vi "Message Window Dialog Box.vi"(4 "parent window name (\"\")":string, 5 "sound? (F)":bool, 6 "modality (0)":i32(ring) items=["Application", "System", "Task"], 7 "icon (0:None)":i32(ring), 8 "buttons (0:OK)":i32(ring), 9 "message (\"\")":string, 10 "window title (\"\")":string) -> (3 "button pressed":i32(ring) items=["OK", "CANCEL", "ABORT", "RETRY", "IGNORE", "YES", "NO"])   [LabVIEW 2011]
doc: "This VI calls the Windows functions MessageBox and MessageBeep to display a message dialog box and, optionally, play a sound effect. These functions are in the Windows DLL called USER.EXE, which is located in the windows\\system directory. If your computer is not equipped with a sound driver, a short \"beep\" will be played through the PC's speaker.\n\nVarious combinations of dialog boxes are possible. The buttons input selects which buttons are displayed in the dialog box, the icon input determines the icon, if any, and the modality box determines whether the dialog box is system, application, or task modal.\n\nThe following dialog box button schemes are available through the \"buttons\" input:\n0: OK\n1: OK / Cancel\n2: Abort / Retry / Ignore\n3: Yes / No / Cancel\n4: Yes / No\n5: Retry / Cancel\n\nThe following icons are available through the \"icon\" input:\n0: None\n1: STOP icon\n2: Question icon\n3: Exclamation icon\n4: Information icon\n\nThe following three modalities are available:\n0: Application\n1: System\n2: Task\n\nIf sounds are enabled, the icon option determines the sound effect played, as defined in the Sounds section of Windows' Control Panel.\n\nThe DLL functions called are:\n\nint MessageBox ( hWndParent, lpText, lpCaption, wType )\nvoid MessageBeep ( wType )\n\nFunction definitions are from:\nMicrosoft Windows Programmer's Reference\nCopyright 1990 Microsoft Corporation."
uses:
  user32.dll
panel:
  in  "buttons":i32[](array[numeric])=[0, 1, 2, 3, 4, 5, 16, 32, 48, 64] format="%.0x"
  in  "icons":i32[](array[numeric])=[0, 16, 32, 48, 64, 5, 16, 32, 48, 64] format="%.0x"
  in  "modal constants":i32[](array[numeric])=[0, 4096, 8192] format="%.0x"
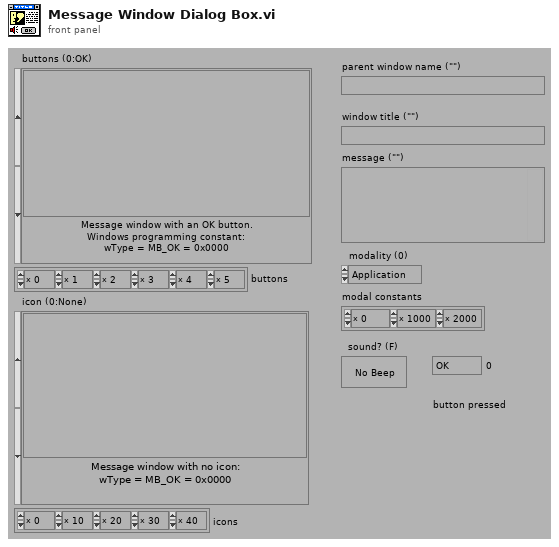
[diagram p1: front panel]
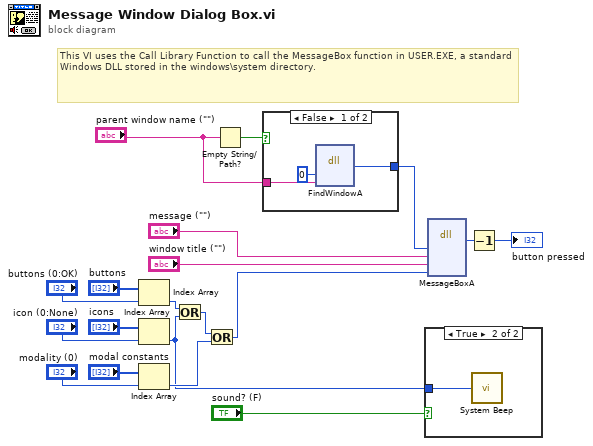
[diagram p0: block diagram]
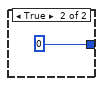
[diagram p2: hidden frame]
diagram:
  # "This VI uses the Call Library Function to call the MessageBox function in USER.EXE, a standard Windows DLL stored in the windows\\system directory."
  n1 = Index Array(array="buttons", index="buttons (0:OK)") -> (element=w7:i32)
  n2 = Index Array(array="icons", index="icon (0:None)") -> (element=w4:i32)
  n3 = Index Array(array="modal constants", index="modality (0)") -> (element=w6:i32)
  n4 = Or(x=w7, y=w4) -> (x .or. y?=w5:i32)
  n5 = Or(x=w5, y=w6) -> (x .or. y?=w11:i32)
  n6 = Empty String/Path?(string/path="parent window name (\"\")") -> (empty?=w2:bool)
  n7 = case shown="False" w2 {
    tunnel: [w21 u32 0] -> w3
    tunnel: "parent window name (\"\")" -> [w20 _]
    frame False {
      n8 = dll-call lib="User32.dll" fn="FindWindowA" label="FindWindow"("lpszClassName"=0, "lpszWindowName"=w20) -> ("hWnd"=w21:u32)  [unwired: 5 in, 2 out]
    }
    frame True {
    }
  }
  n9 = case shown="True" "sound? (F)" {
    tunnel: w4 -> [_ w24]
    frame False {
      # "Do not play sound effects."
    }
    frame True {
      n10 = call "System Beep.vi"("icon (0:None)"=w24) -> ()  [unwired: 1 out]
    }
  }
  n11 = dll-call lib="User32.dll" fn="MessageBoxA" label="MessageBox"("hWndParent"=w3, "lpText"="message (\"\")", "lpCaption"="window title (\"\")", "wType"=w11) -> (w16:i32)  [unwired: 7 in, 2 out]
  n12 = Decrement(x=w16) -> (x-1=→"button pressed":i32)
